vi "problem_1.vi"() -> ()   [LabVIEW 2020]
panel:
  in  "Total Time in Seconds":dbl
  out "Seconds":dbl
  out "Minutes":dbl
  out "Hours":dbl
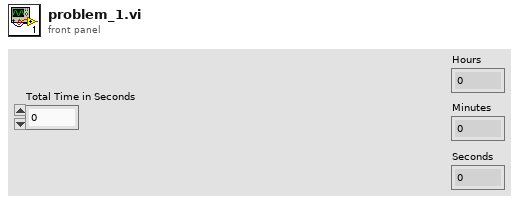
[diagram p1: front panel]
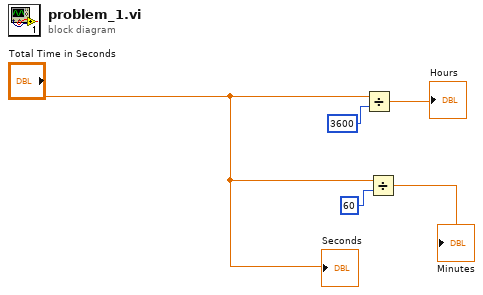
[diagram p0: block diagram]
diagram:
  n1 = Divide(x="Total Time in Seconds", y=3600) -> (x/y=→"Hours":dbl)
  n2 = Divide(x="Total Time in Seconds", y=60) -> (x/y=→"Minutes":dbl)
  "Seconds" <- "Total Time in Seconds"
